vi "1A Steven's Defilter.vi"(3 "Angle?(F)":bool, 4 "# to running average":i32=3, 5 "Value In":dbl) -> (2 "Filtered Value Out":dbl)   [LabVIEW 2011]
doc: "The airmar sensor has a filter built in to it which slows down the response time of the sensor to changes.\nSteven Zhang designed this de-filter to counter this.\nUsing this VI will introduce more noise but should give a quicker response time.\nif \"Angle?\" input is True, input will be appropriately unwrapped and rewrapped to a 0-to-360-degree range."
uses:
  <vilib>/Analysis/3filter.llb/FIR Filter (DBL).vi
  <vilib>/ptbypt/NI_PtbyPt.lvlib
  <vilib>/Analysis/NI_AALBase.lvlib
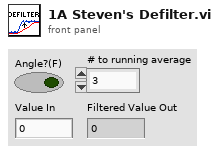
[diagram p1: front panel]
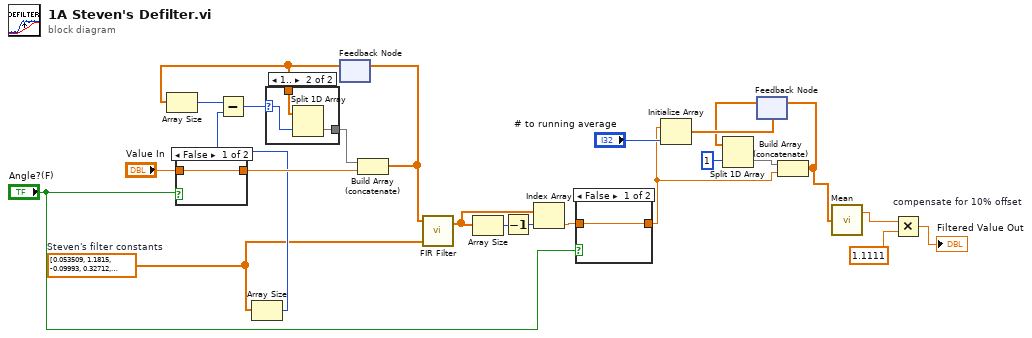
[diagram p0: block diagram]
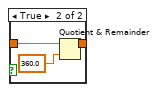
[diagram p2: hidden frame]
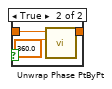
[diagram p3: hidden frame]
diagram:
  w10 = dbl[] [0.053509, 1.1815, -0.09993, 0.32712, 0.10938, 0.11358, 0.13924, -0.16172, 0.45069, -0.055441, 0.019471, 0.082764, 0.12364, -0.39235, -0.19677, 0.3546, 0.16406, -0.070202, -0.10287, -0.028649, 0.018791, -0.038948, 0.097859, -0.0038871, -0.027341, 0.025466, 0.10393, -0.25443, 0.039379, -0.052109, -0.089114, 0.018497, -0.76719, 0.10647, -0.024919, -0.062391, 0.024126, 0.47711, -1.0783, 0.17365, 0.32185, 0.30825, 0.069773, 0.0316, -0.81283, -0.038254, 0.1407, 0.043989, 0.064417, 0.051313, 0.19402, -0.16605]  # Steven's filter constants
  n1 = case shown="False" "Angle?(F)" {
    tunnel: [w25 w27] -> w24
    tunnel: "Value In" -> [w25 w26]
    frame False {
    }
    frame True {
      n2 = call <vilib>:"Unwrap Phase PtByPt.vi"("wrap base"=360.0, "phase"=w26) -> ("unwrapped phase"=w27:dbl)  [unwired: 9 in]
    }
  }
  n3 = Array Size(array=w10) -> (size(s)=w15:i32)
  n4 = feedback #1() -> (w18:dbl[])  [unwired: 1 in]
  n5 = Array Size(array=w18) -> (size(s)=w16:i32)
  n6 = Subtract(x=w16, y=w15) -> (x-y=w17:i32)
  n7 = case shown="1.." w17 {
    selector: w17 -> [_ w30]
    tunnel: [w29 w32] -> w23
    tunnel: w18 -> [w29 w31]
    frame 0, Default {
    }
    frame 1.. {
      n8 = Split 1D Array(array=w31, index=w30) -> (second subarray=w32:dbl[])  [unwired: 1 out]
    }
  }
  n9 = Build Array (concatenate)(w23, w24) -> (w22:dbl[])
  n10 = feedback-in #1(w22) -> ()
  n11 = call-poly <vilib>:"FIR Filter.vi"("FIR Coefficients"=w10, "X"=w22) -> ("Filtered X"=w20:dbl[])  [unwired: 2 in, 1 out]
  n12 = Array Size(array=w20) -> (size(s)=w21:i32)
  n13 = Decrement(x=w21) -> (x-1=w9:i32)
  n14 = Index Array(array=w20, index=w9) -> (element=w14:dbl)
  n15 = case shown="False" "Angle?(F)" {
    tunnel: w14 -> [w33 w36]
    tunnel: [w33 w35] -> w5
    frame False {
    }
    frame True {
      n16 = Quotient & Remainder(x=w36, y=360.0) -> (x-y*floor(x/y)=w35:dbl)  [unwired: 1 out]
    }
  }
  n17 = Initialize Array(w5, "# to running average") -> (w4:dbl[])
  n18 = feedback #2(w4) -> (w3:dbl[])
  n19 = Split 1D Array(array=w3, index=1) -> (second subarray=w6:dbl[])  [unwired: 1 out]
  n20 = Build Array (concatenate)(w6, w5) -> (w1:dbl[])
  n21 = feedback-in #2(w1) -> ()
  n22 = call <vilib>:"Mean.vi"("X"=w1) -> ("mean"=w2:dbl)  [unwired: 1 out]
  n23 = Multiply "compensate for 10% offset"(x=w2, y=1.1111) -> (x*y=→"Filtered Value Out":dbl)
